vi "Build Preview.vi"(7 "Ambient":dbl, 8 "error in (no error)":errorcluster, 9 "Start Temp":dbl, 10 "Start Time":dbl, 11 "Rate Step in":refnum<class "Rate Step.lvclass">) -> (0 "error out":errorcluster, 1 "End Temp":dbl, 2 "End Time":dbl, 3 "Rate Step out":refnum<class "Rate Step.lvclass">, 4 "Step Plot Data":cluster{"Time":dbl[], "Value":dbl[]})   [LabVIEW 2018, in "Temp Recipe.lvlib" / "Rate Step.lvclass"]
uses:
  Rate Step.lvclass
  Rate Step.lvclass/Rate Step.ctl
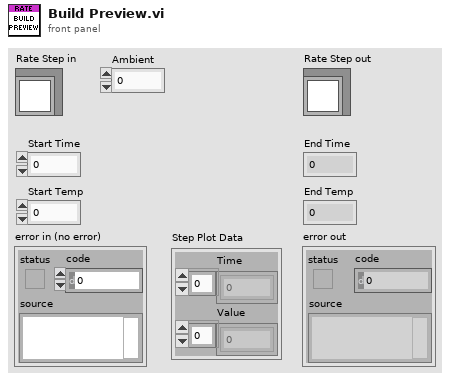
[diagram p1: front panel]
types:
  T1 = typedef "Temp Recipe.lvlib/Rate Step.lvclass/Ref Data.ctl" = cluster{"Step Temp":dbl, "Step Time":dbl, "Target":dbl}
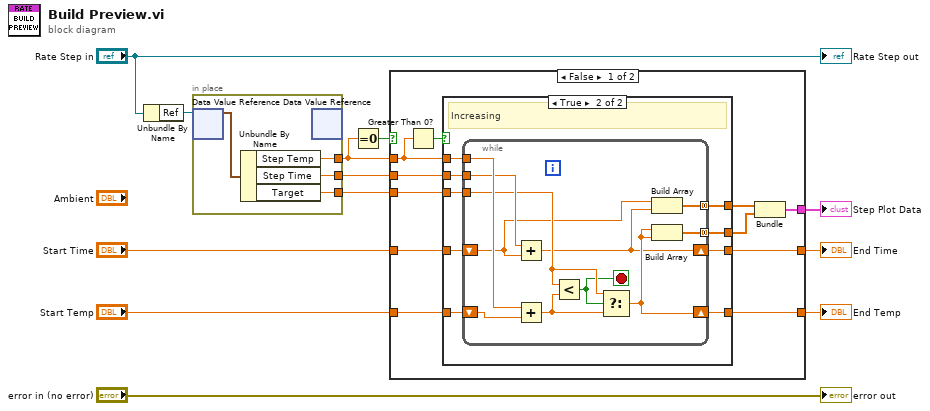
[diagram p0: block diagram]
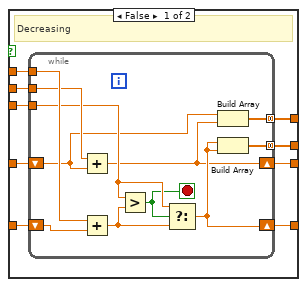
[diagram p2: hidden frame]
diagram:
  n1 = Unbundle By Name("Rate Step in") -> ("Ref"=w11:refnum<data-value>)
  n2 = in-place {
    in-place-border: [w15] -> w7
    in-place-border: [w14] -> w9
    in-place-border: [w13] -> w8
    n3 = in-place-dvr #1(w11) -> (w16:T1)  [unwired: 1 out]
    n4 = Unbundle By Name(w16) -> ("Step Temp"=w15:dbl, "Step Time"=w14:dbl, "Target"=w13:dbl)
    n5 = in-place-dvr #1() -> ()  [unwired: 1 in, 2 out]
  }
  n6 = Equal To 0?(x=w7) -> (x = 0?=w6:bool)
  n7 = case shown="False" w6 {
    tunnel: w7 -> [w26 _]
    tunnel: w9 -> [w25 _]
    tunnel: w8 -> [w24 _]
    tunnel: "Start Time" -> [w23 w69]
    tunnel: "Start Temp" -> [w22 w68]
    tunnel: [w21 w68] -> w3
    tunnel: [w20 w69] -> w2
    tunnel: [w17 _] -> w1
    frame False {
      n8 = Greater Than 0?(x=w26) -> (x > 0?=w27:bool)
      n9 = case shown="True" w27 {
        tunnel: w26 -> [w32 w52]
        tunnel: w25 -> [w31 w51]
        tunnel: w24 -> [w30 w50]
        tunnel: w23 -> [w36 w56]
        tunnel: w22 -> [w35 w55]
        tunnel: [w34 w54] -> w21
        tunnel: [w33 w53] -> w20
        tunnel: [w29 w49] -> w19
        tunnel: [w28 w48] -> w18
        frame False {
          # "Decreasing"
          n10 = while {
            shift-right: [w40] -> w34
            shift-left: w35 -> [w47]
            shift-right: [w38] -> w33
            shift-left: w36 -> [w39]
            tunnel: w32 -> [w46]
            tunnel: w31 -> [w45]
            tunnel: w30 -> [w43]
            tunnel: [w41] -> w28 mode=concatenating
            tunnel: [w37] -> w29 mode=concatenating
            stop <- w42 stop-if-true
            n11 = Add(x=w45, y=w39) -> (x+y=w38:dbl)
            n12 = Add(x=w46, y=w47) -> (x+y=w44:dbl)
            n13 = Greater?(x=w43, y=w44) -> (0:w42:bool)
            n14 = Select(t=w43, s=w42, f=w44) -> (s? t:f=w40:dbl)
            n15 = Build Array(w39, w38) -> (w37:dbl[])
            n16 = Build Array(w40, w40) -> (w41:dbl[])
          }
        }
        frame True {
          # "Increasing"
          n17 = while {
            shift-right: [w60] -> w54
            shift-left: w55 -> [w67]
            shift-right: [w58] -> w53
            shift-left: w56 -> [w59]
            tunnel: w52 -> [w66]
            tunnel: w51 -> [w65]
            tunnel: w50 -> [w63]
            tunnel: [w61] -> w48 mode=concatenating
            tunnel: [w57] -> w49 mode=concatenating
            stop <- w62 stop-if-true
            n18 = Add(x=w65, y=w59) -> (x+y=w58:dbl)
            n19 = Add(x=w66, y=w67) -> (x+y=w64:dbl)
            n20 = Less?(x=w63, y=w64) -> (x < y?=w62:bool)
            n21 = Select(t=w63, s=w62, f=w64) -> (s? t:f=w60:dbl)
            n22 = Build Array(w59, w58) -> (w57:dbl[])
            n23 = Build Array(w60, w60) -> (w61:dbl[])
          }
        }
      }
      n24 = Bundle(w19, w18) -> (w17:cluster{dbl[], dbl[]})  [unwired: 1 in]
    }
    frame True {
      # "Prevent Infinite Loop\n\nIRL, you would do something more noticeable than just skipping the step."
    }
  }
  "Step Plot Data" <- w1
  "End Time" <- w2
  "End Temp" <- w3
  "error out" <- "error in (no error)"
  "Rate Step out" <- "Rate Step in"
